vi "Set Trigger Count.vi"(8 "error in":errorcluster, 10 "Count":dbl min=0.0 max=9999.0 step=1.0, 11 "VISA resource name in":refnum<visa-resource-name>) -> (0 "error out":errorcluster, 3 "VISA resource name out":refnum<visa-resource-name>)   [LabVIEW 2021, in "Keysight U1282A.lvlib"]
doc: "El comando de definir el contador de disparo (TRIG:REF:COUN) se utiliza para establecer el conteo del modo auto hold."
uses:
  Keysight U1282A.lvlib
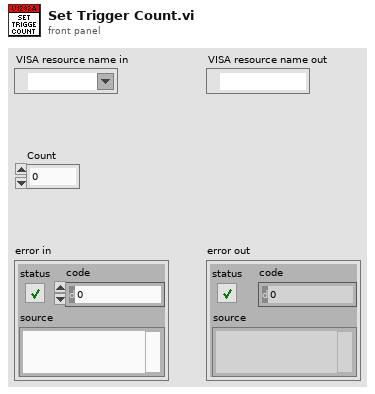
[diagram p1: front panel]
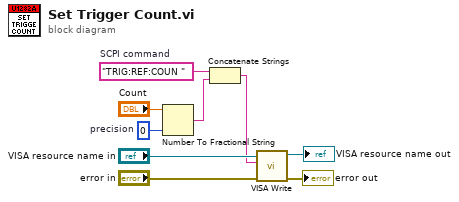
[diagram p0: block diagram]
diagram:
  w3 = "TRIG:REF:COUN "  # SCPI command
  w4 = i16 0  # precision
  n1 = Number To Fractional String(number="Count", precision (6)=w4) -> (F-format string=w2:string)  [unwired: 2 in]
  n2 = Concatenate Strings(w3, w2) -> (w1:string)
  n3 = call "VISA Write.vi"("error in"="error in", "SCPI command"=w1, "VISA resource in"="VISA resource name in") -> ("error out"=→"error out":errorcluster, "VISA resource out"=→"VISA resource name out":refnum<visa-resource-name>)  [unwired: 6 in, 1 out]
